vi "One Dynamic Input No Dynamic Output.vi"(8 "error in (no error)":errorcluster, 11 "Class Gamma in":refnum<class "Class Gamma.lvclass">) -> (0 "error out":errorcluster, 1 "Class Alpha out":refnum<class "Class Alpha.lvclass">)   [LabVIEW 2023, in "Class Gamma.lvclass"]
doc: "This VI overrides the VI of the same name in Class Alpha."
uses:
  Class Gamma.lvclass
  Class Alpha/Class Alpha.lvclass
  c:/dev/_r/4/eng/lv-core/lvpostprocessingd/lv_mc_x86_64/dist_i386/examples/Object-Oriented Programming/Dynamic Terminals/Class Alpha/Class Alpha.lvclass
  Class Gamma.lvclass/Class Gamma.ctl
  Class Beta/Class Beta.lvclass
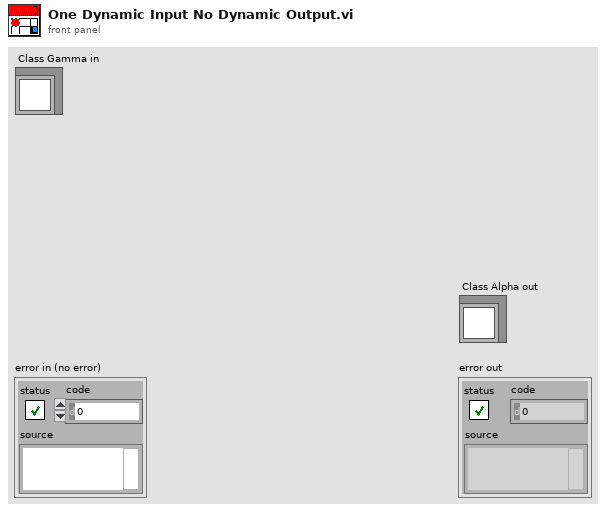
[diagram p1: front panel]
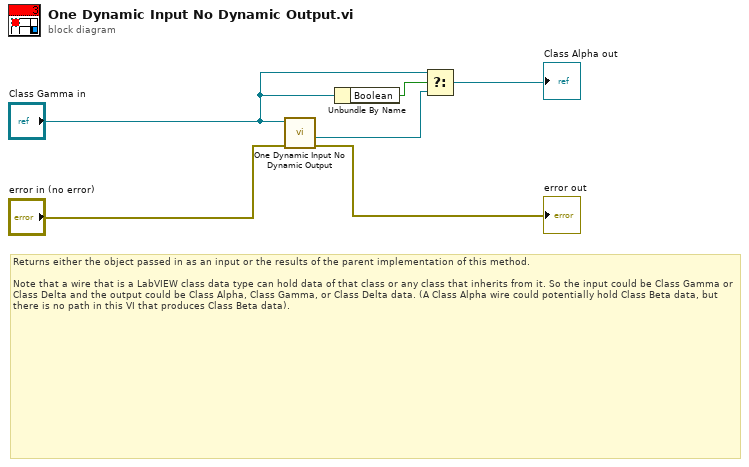
[diagram p0: block diagram]
diagram:
  # "Returns either the object passed in as an input or the results of the parent implementation of this method.\n\nNote that a wire that is a LabVIEW class data type can hold data of that class or any class that inherits from it. So the input could be Class Gamma or Class Delta and the output could be Class Alpha, Class Gamma, or Class Delta data. (A Class Alpha wire could potentially hold Class Beta data, but there is no path in this VI that produces Class Beta data)."
  n1 = call-parent "One Dynamic Input No Dynamic Output.vi"("error in (no error)"="error in (no error)", "Class Alpha in"="Class Gamma in") -> ("error out"=→"error out":errorcluster, "Class Alpha out"=w4:refnum<class "Class Alpha.lvclass">)  [unwired: 8 in]
  n2 = Unbundle By Name("Class Gamma in") -> ("Boolean"=w1:bool)
  n3 = Select(t="Class Gamma in", s=w1, f=w4) -> (s? t:f=→"Class Alpha out":refnum<class "Class Alpha.lvclass">)
